vi "Drive PID.vi"(8 "Wait Length":i32, 9 "Angle":dbl, 10 "Distance":dbl, 11 "drive in":T18) -> (2 "In Range?":bool, 3 "drive out":T18)   [LabVIEW 2014]
uses:
  <vilib>/Rock Robotics/WPI/RobotDrive/WPI_RobotDriveDevRef.ctl
  <vilib>/Rock Robotics/WPI/MotorControl/WPI_MotorControlDeviceRef.ctl
  <vilib>/Rock Robotics/WPI/MotorControl/WPI_MotorControlType.ctl
  <vilib>/Rock Robotics/SystemInterfaces/Typedef/FPGA_TypedefDigitalModule.ctl
  <vilib>/Rock Robotics/SystemInterfaces/DIO/FPGA_DIOPWMChannel.ctl
  <vilib>/Rock Robotics/WPI/PWM/WPI_PWMDeadband.ctl
  <vilib>/Rock Robotics/WPI/CAN/Jaguar/SubVIs/WPI_CANJaguar_ControlMode.ctl
  <vilib>/Rock Robotics/WPI/CAN/TalonSRX/WPI_CANTalonSRX_APIControlMode.ctl
  <vilib>/Rock Robotics/WPI/PWM/WPI_PWMTransform_ConPane.ctl
  <vilib>/Rock Robotics/WPI/Encoder/WPI_EncoderDevRef.ctl
  <vilib>/Rock Robotics/SystemInterfaces/Encoder/FPGA_EncoderIdx.ctl
  <vilib>/Rock Robotics/SystemInterfaces/Counter/FPGA_CounterCtrSystemIndex.ctl
  <vilib>/Rock Robotics/WPI/Encoder/WPI_EncoderType.ctl
  <vilib>/Rock Robotics/WPI/Gyro/WPI_GyroDevRef.ctl
  <vilib>/Rock Robotics/SystemInterfaces/Typedef/FPGA_TypedefAnalogModule.ctl
  <vilib>/Rock Robotics/SystemInterfaces/AI/FPGA_AIChannel.ctl
  <vilib>/Rock Robotics/WPI/RobotDrive/WPI_RobotDriveArcadeDrive_Standard(NoSaturation).vi
panel:
  in  "turn dead band":dbl
  in  "straight dead band":dbl
  in  "turn gains":cluster{"P":dbl, "I":dbl, "D":dbl}
  in  "straight gains":cluster{"P":dbl, "I":dbl, "D":dbl}
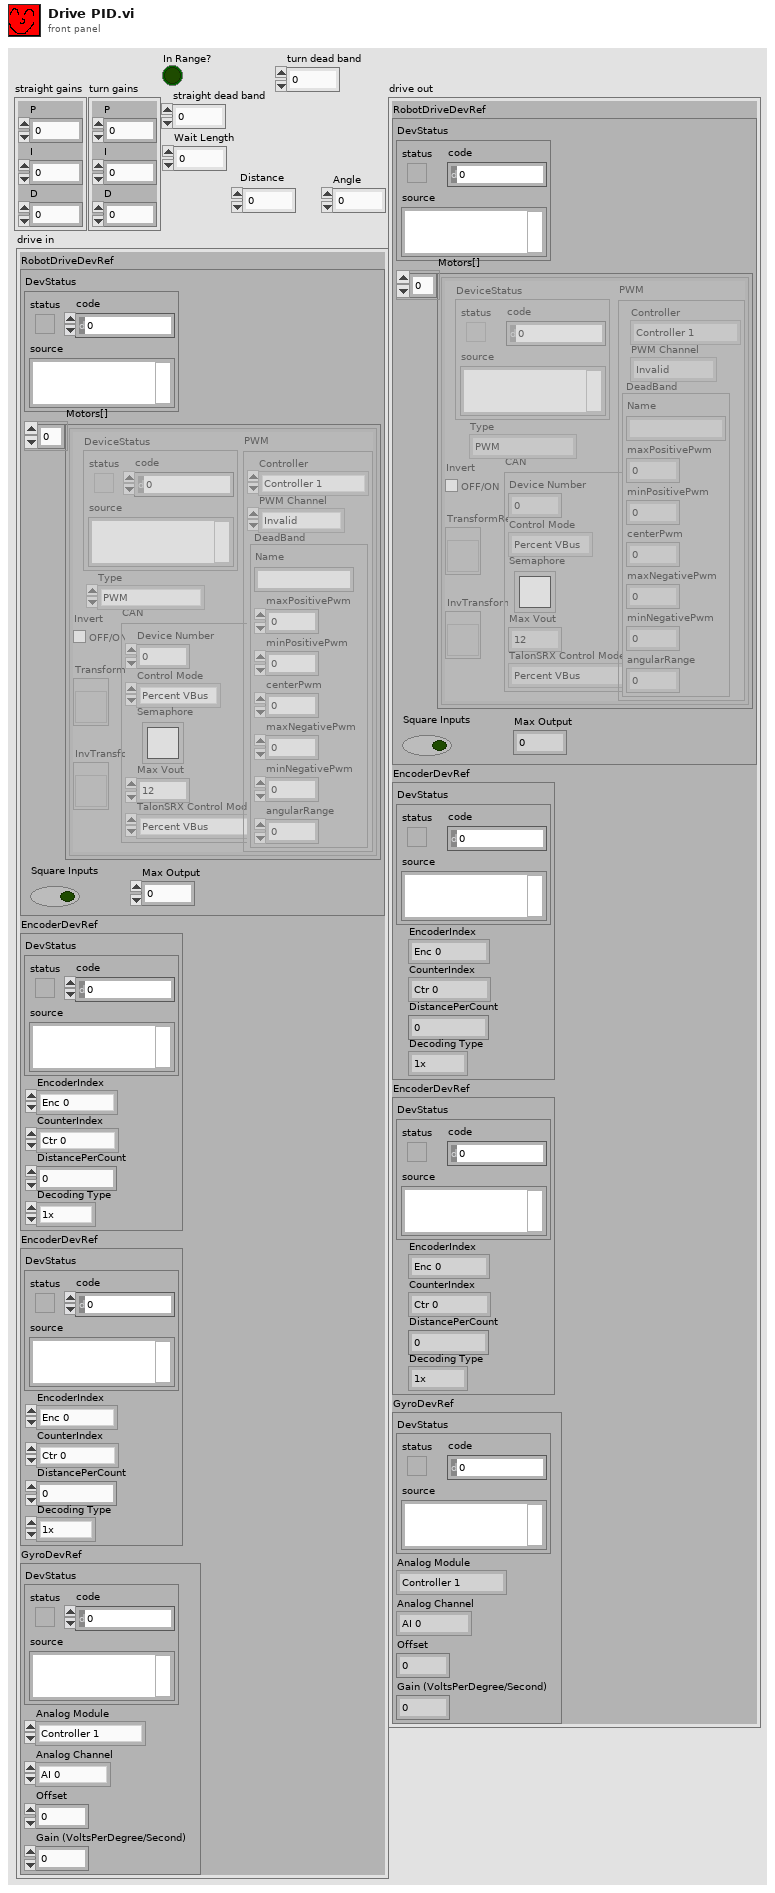
[diagram p1: front panel]
types:
  T1 = typedef "WPI_RobotDriveDevRef.ctl" = cluster{"DevStatus":errorcluster, "Motors[]":T2[], "Square Inputs":bool, "Max Output":dbl}
  T2 = typedef "WPI_MotorControlDeviceRef.ctl" = cluster{"DeviceStatus":errorcluster, "Type":T3, "PWM":cluster{"Controller":T4, "PWM Channel":T5, "DeadBand":T6}, "CAN":cluster{"Device Number":u8, "Control Mode":T7, "Semaphore":T8, "Max Vout":dbl, "TalonSRX Control Mode":T9}, "Invert":bool, "TransformRef":T10, "InvTransformRef":T10}
  T3 = typedef "WPI_MotorControlType.ctl" = enum16{"PWM", "CAN", "CANTalonSRX"}
  T4 = typedef "FPGA_TypedefDigitalModule.ctl" = enum16{"Controller 1"}
  T5 = typedef "FPGA_DIOPWMChannel.ctl" = enum8{"PWM 0", "PWM 1", "PWM 2", "PWM 3", "PWM 4", "PWM 5", "PWM 6", "PWM 7", "PWM 8", "PWM 9", "PWM MXP 0", "PWM MXP 1", "PWM MXP 2", "PWM MXP 3", "PWM MXP 4", "PWM MXP 5", "PWM MXP 6", "PWM MXP 7", "PWM MXP 8", "PWM MXP 9", "Invalid"}
  T6 = typedef "WPI_PWMDeadband.ctl" = cluster{"Name":string, "maxPositivePwm":i32, "minPositivePwm":i32, "centerPwm":i32, "maxNegativePwm":i32, "minNegativePwm":i32, "angularRange":u16}
  T7 = typedef "WPI_CANJaguar_ControlMode.ctl" = enum8{"Percent VBus", "Current", "Speed", "Position", "Voltage"}
  T8 = typedef "Semaphore RefNum" = refnum<k1>
  T9 = typedef "WPI_CANTalonSRX_APIControlMode.ctl" = enum8{"Percent VBus", "Speed", "Position", "Slave", "Unchanged / Invalid"}
  T10 = typedef "WPI_PWMTransform_ConPane.ctl" = refnum<vi>
  T11 = typedef "WPI_EncoderDevRef.ctl" = cluster{"DevStatus":errorcluster, "EncoderIndex":T12, "CounterIndex":T13, "DistancePerCount":dbl, "Decoding Type":T14}
  T12 = typedef "FPGA_EncoderIdx.ctl" = enum8{"Enc 0", "Enc 1", "Enc 2", "Enc 3", "Enc 4", "Enc 5", "Enc 6", "Enc 7", "Invalid"}
  T13 = typedef "FPGA_CounterCtrSystemIndex.ctl" = enum8{"Ctr 0", "Ctr 1", "Ctr 2", "Ctr 3", "Ctr 4", "Ctr 5", "Ctr 6", "Ctr 7", "Invalid"}
  T14 = typedef "WPI_EncoderType.ctl" = enum16{"1x", "2x", "4x"}
  T15 = typedef "WPI_GyroDevRef.ctl" = cluster{"DevStatus":errorcluster, "Analog Module":T16, "Analog Channel":T17, "Offset":dbl, "Gain (VoltsPerDegree/Second)":dbl}
  T16 = typedef "FPGA_TypedefAnalogModule.ctl" = enum16{"Controller 1"}
  T17 = typedef "FPGA_AIChannel.ctl" = enum8{"AI 0", "AI 1", "AI 2", "AI 3", "AI MXP 0", "AI MXP 1", "AI MXP 2", "AI MXP 3", "Invalid"}
  T18 = cluster{"RobotDriveDevRef":T1, "EncoderDevRef":T11, "EncoderDevRef":T11, "GyroDevRef":T15}
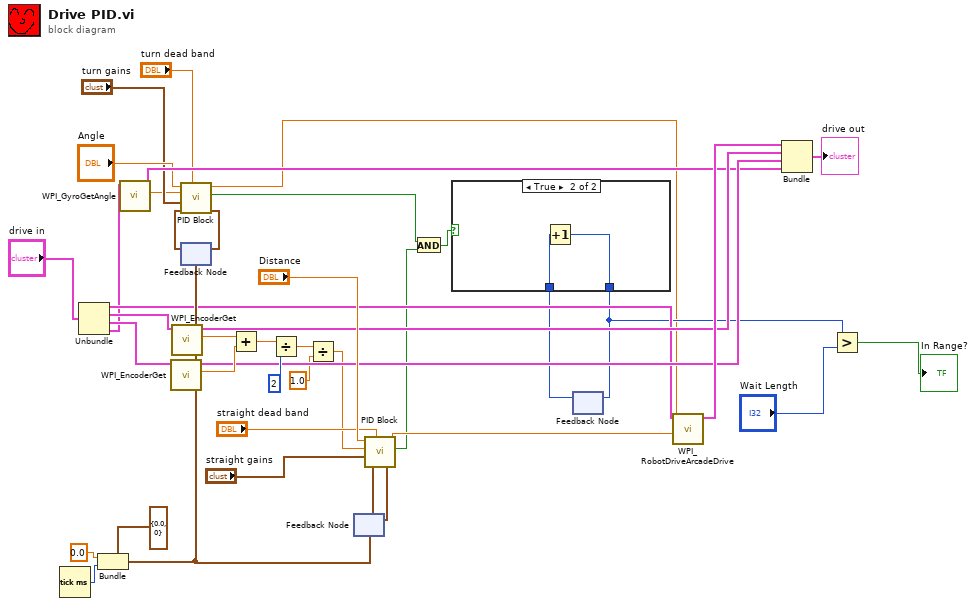
[diagram p0: block diagram]
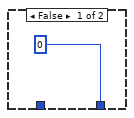
[diagram p2: hidden frame]
diagram:
  n1 = Tick Count (ms)() -> (millisecond timer value=w31:u32)
  n2 = Unbundle("drive in") -> ("RobotDriveDevRef"=w22:T1, "EncoderDevRef"=w21:T11, "EncoderDevRef"=w20:T11, "GyroDevRef"=w19:T15)
  n3 = Bundle(cluster=cluster{"Last Error":dbl, "Last Time":u32} {"Last Error"=0.0, "Last Time"=0} ("To Shift"), "Last Error"=0.0, "Last Time"=w31) -> (w30:cluster{"Last Error":dbl, "Last Time":u32})
  n4 = call <vilib>:"WPI_GyroGetAngle.vi"("GyroDevRef"=w19) -> ("Angle"=w4:dbl, "GyroDevRef"=w25:T15)  [unwired: 7 in, 2 out]
  n5 = call <vilib>:"WPI_EncoderGet.vi"("EncoderDevRef"=w20) -> ("Distance"=w41:dbl, "EncoderDevRef"=w26:T11)  [unwired: 5 in, 4 out]
  n6 = call <vilib>:"WPI_EncoderGet.vi"("EncoderDevRef"=w21) -> ("Distance"=w40:dbl, "EncoderDevRef"=w27:T11)  [unwired: 5 in, 4 out]
  n7 = feedback #1(w30) -> (w8:cluster{"Last Error":dbl, "Last Time":u32})
  n8 = call "PID Block.vi"("Deadband"="turn dead band", "From Shift"=w8, "Gains"="turn gains", "Position"=w4, "Setpoint"="Angle") -> ("To Shift"=w7:cluster{"Last Error":dbl, "Last Time":u32}, "Tolerable?"=w6:bool, "Output"=w5:dbl)  [unwired: 4 in]
  n9 = feedback-in #1(w7) -> ()
  n10 = Add(x=w40, y=w41) -> (x+y=w39:dbl)
  n11 = Divide(x=w39, y=2) -> (x/y=w3:dbl)
  n12 = Divide(x=w3, y=1.0) -> (x/y=w2:dbl)
  n13 = feedback #2(w30) -> (w34:cluster{"Last Error":dbl, "Last Time":u32})
  n14 = call "PID Block.vi"("Deadband"="straight dead band", "From Shift"=w34, "Gains"="straight gains", "Position"=w2, "Setpoint"="Distance") -> ("To Shift"=w35:cluster{"Last Error":dbl, "Last Time":u32}, "Tolerable?"=w18:bool, "Output"=w29:dbl)  [unwired: 4 in]
  n15 = feedback-in #2(w35) -> ()
  n16 = And(x=w6, y=w18) -> (x .and. y?=w16:bool)
  n17 = feedback #3() -> (w15:i32)  [unwired: 1 in]
  n18 = case shown="True" w16 {
    tunnel: [0 w44] -> w14
    tunnel: w15 -> [_ w43]
    frame False {
    }
    frame True {
      n19 = Increment(x=w43) -> (x+1=w44:i32)
    }
  }
  n20 = feedback-in #3(w14) -> ()
  n21 = call-poly <vilib>:"WPI_RobotDriveArcadeDrive.vi"("Y axis value"=w29, "X axis value"=w5, "RobotDriveDevRef"=w22) -> ("RobotDriveDevRef"=w28:T1)  [unwired: 6 in, 2 out]
  n22 = Bundle("RobotDriveDevRef"=w28, "EncoderDevRef"=w27, "EncoderDevRef"=w26, "GyroDevRef"=w25) -> (→"drive out":T18)  [unwired: 1 in]
  n23 = Greater?(x=w14, y="Wait Length") -> (0:→"In Range?":bool)
